vi "SVG Scale Example.vi"() -> ()   [LabVIEW 2020]
doc: "G-Image example demonstrating loading a vector image with adjustable scaling."
uses:
  <vilib>/picture/picture.llb/imagedata.ctl
  <vilib>/Utility/miscctls.llb/LVPointTypeDef.ctl
  Image IO/Polymorphic VIs/Load SVG Image (Path).vi
  <vilib>/Utility/cursorutil.llb/Set Cursor (Icon Pict).vi
  G-Image.lvlib
panel:
  in  "Reset View":bool
  in  "Image":u16(ring) items=["vector-gradient.svg", "vector.svg"]
  in  "Stop":bool
  out "2D Picture":picture
  in  "Scale":dbl(slide)=1.0 min=0.1 max=4.0 step=0.1 scale=0.1..4.0
  # "Instructions:\n1. Run the VI.\n2. Select a vector image to scale from the Image ring. \n3. Adjust the Scale slider to change the size of the vector image as it is loaded.\n4. Click and drag the image to pan the view. Reset the view by clicking Reset View."
  # "G"
  # "-Image"
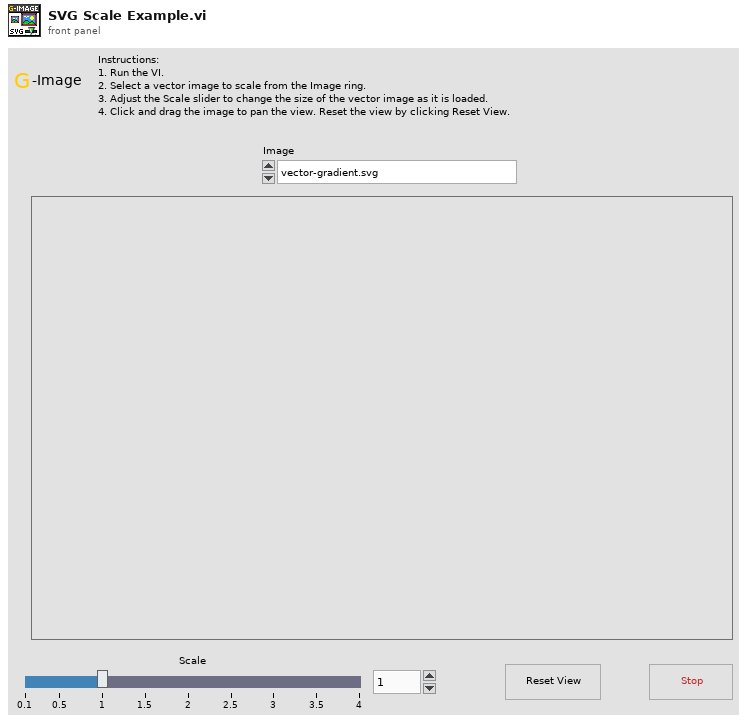
[diagram p1: front panel]
types:
  T1 = typedef "imagedata.ctl" = cluster{"image type":i32, "image depth":i32, "image":u8[], "mask":u8[], "colors":u32[], "Rectangle":cluster{"left":i16, "top":i16, "right":i16, "bottom":i16}}
  T2 = typedef "LVPoint32TypeDef.ctl" = cluster{"Horizontal":i32, "Vertical":i32}
  T3 = typedef "LVPointTypeDef.ctl" = cluster{"Horizontal":i16, "Vertical":i16}
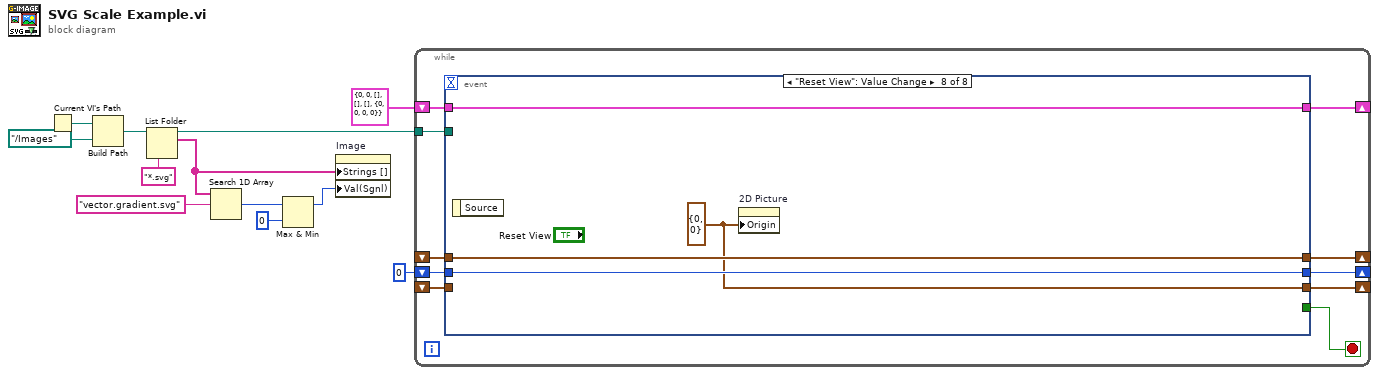
[diagram p0: block diagram]
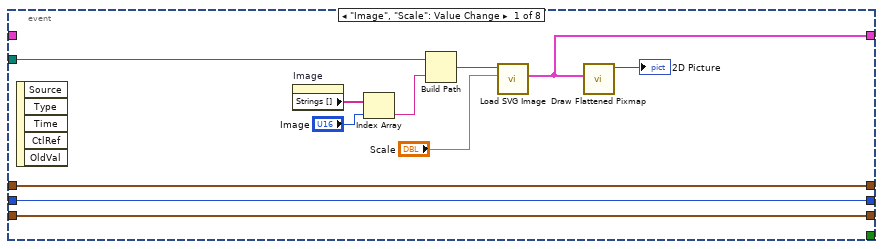
[diagram p2: hidden frame]
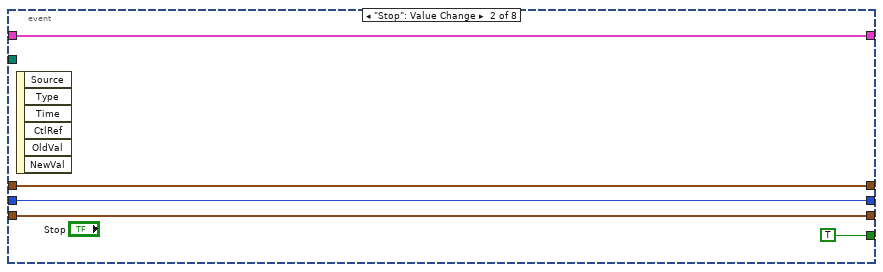
[diagram p3: hidden frame]
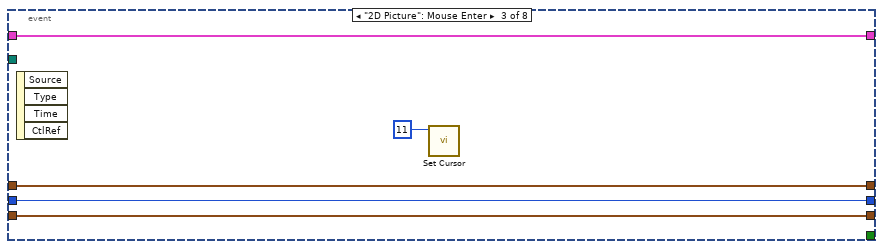
[diagram p4: hidden frame]
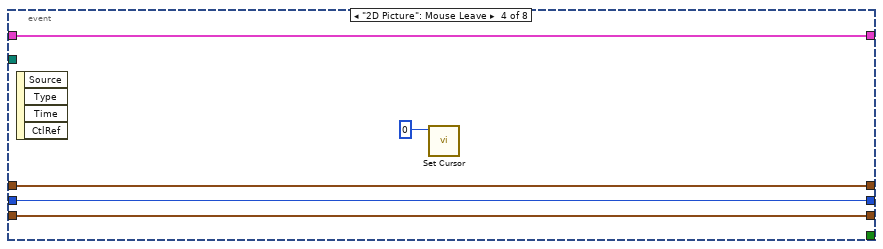
[diagram p5: hidden frame]
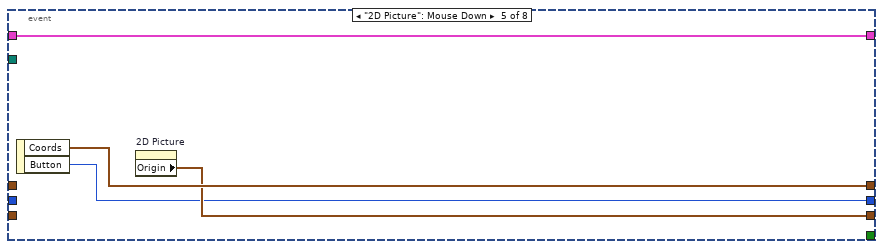
[diagram p6: hidden frame]
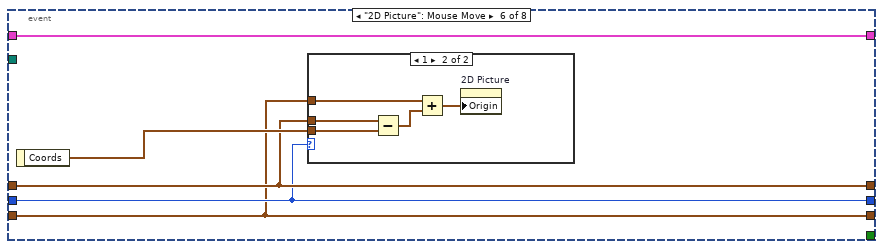
[diagram p7: hidden frame]
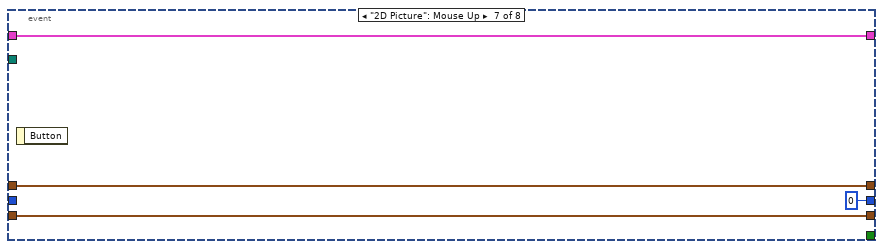
[diagram p9: hidden frame]
diagram:
  n1 = Current VI's Path() -> (path=w12:path)
  n2 = Build Path(base path=w12, name or relative path=path "../Images") -> (appended path=w10:path)
  n3 = List Folder(path=w10, pattern="*.svg") -> (path out=w9:path, filenames=w7:string[])  [unwired: 2 in, 2 out]
  n4 = Search 1D Array(1D array=w7, element="vector.gradient.svg") -> (index of element=w5:i32)  [unwired: 1 in]
  n5 = Max & Min(x=w5, y=0) -> (max(x,y)=w3:i32)  [unwired: 1 out]
  n6 = property on="Image" class="Ring (strict)"("Strings []"=w7, "Val(Sgnl)"=w3) -> ()  [unwired: 2 in, 2 out]
  n7 = while {
    tunnel: w9 -> [w20]
    shift-right: [w19] -> _
    shift-left: T1 {"image type"=0, "image depth"=0, "image"=[], "mask"=[], "colors"=[], "Rectangle"={"left"=0, "top"=0, "right"=0, "bottom"=0}} ("Image") -> [w22]
    shift-right: [w18] -> _
    shift-left: _ -> [w14]
    shift-right: [w17] -> _
    shift-left: _ -> [w16]
    shift-right: [w15] -> _
    shift-left: u16 0 ("Button") -> [w13]
    stop <- w21 stop-if-true
    n8 = event shown="[7] \"Reset View\": Value Change" {
      selector: _ -> [_ _ _ _ _ _ _ _]
      dyn-events: _ -> [_ _ _ _ _ _ _ _]
      timeout: _ -> [_ _ _ _ _ _ _ _]
      tunnel: w22 -> [_ w37 w42 w47 w49 w53 w66 w70]
      tunnel: [_ TRUE _ _ _ _ _ _] -> w21
      tunnel: w20 -> [w33 _ _ _ _ _ _ _]
      tunnel: [w27 w37 w42 w47 w49 w53 w66 w70] -> w19
      tunnel: [w25 w36 w41 w46 w52 w56 w65 w69] -> w18
      tunnel: [w23 w34 w39 w44 w51 w54 w64 w67] -> w17
      tunnel: w16 -> [w23 w34 w39 w44 _ w54 w64 _]
      tunnel: [w24 w35 w40 w45 w50 w55 u16 0 ("Button") w68] -> w15
      tunnel: w14 -> [w25 w36 w41 w46 _ w56 w65 w69]
      tunnel: w13 -> [w24 w35 w40 w45 _ w55 _ w68]
      event "Image", "Scale": Value Change {
        n9 = event-data() -> ()  [unwired: 1 in, 5 out]
        n10 = property on="Image" class="Ring (strict)"() -> ("Strings []"=w32:string[])  [unwired: 2 in, 2 out]
        n11 = Index Array(array=w32, index="Image") -> (element=w30:string)
        n12 = Build Path(base path=w33, name or relative path=w30) -> (appended path=w29:path)
        n13 = call-poly "Load SVG Image.vi"("Scale (1)"="Scale", "Path In"=w29) -> ("Image"=w27:T1)  [unwired: 7 in, 2 out]
        n14 = call <vilib>:"Draw Flattened Pixmap.vi"("image data"=w27) -> ("new picture"=→"2D Picture":picture)  [unwired: 8 in]
      }
      event "Stop": Value Change {
        n15 = event-data() -> ()  [unwired: 1 in, 6 out]
      }
      event "2D Picture": Mouse Enter {
        n16 = event-data() -> ()  [unwired: 1 in, 4 out]
        n17 = call-poly <vilib>:"Set Cursor.vi"("icon"=u16 11) -> ()  [unwired: 9 in, 2 out]
      }
      event "2D Picture": Mouse Leave {
        n18 = event-data() -> ()  [unwired: 1 in, 4 out]
        n19 = call-poly <vilib>:"Set Cursor.vi"("icon"=u16 0) -> ()  [unwired: 9 in, 2 out]
      }
      event "2D Picture": Mouse Down {
        n20 = event-data() -> ("Coords"=w52:T2, "Button"=w50:u16)  [unwired: 1 in]
        n21 = property on="2D Picture" class="Pict"() -> ("Origin"=w51:T3)  [unwired: 2 in, 2 out]
      }
      event "2D Picture": Mouse Move {
        n22 = event-data() -> ("Coords"=w57:T2)  [unwired: 1 in]
        n23 = case shown="1" w55 {
          tunnel: w57 -> [_ w62]
          tunnel: w56 -> [_ w61]
          tunnel: w54 -> [_ w59]
          frame 0, Default {
          }
          frame 1 {
            n24 = Subtract(x=w61, y=w62) -> (x-y=w60:T2)
            n25 = Add(x=w59, y=w60) -> (x+y=w58:T2)
            n26 = property on="2D Picture" class="Pict"("Origin"=w58) -> ()  [unwired: 2 in, 2 out]
          }
        }
      }
      event "2D Picture": Mouse Up {
        n27 = event-data() -> ()  [unwired: 1 in, 1 out]
      }
      event "Reset View": Value Change {
        w67 = T3 {"Horizontal"=0, "Vertical"=0} ("Origin")
        n28 = event-data() -> ()  [unwired: 1 in, 1 out]
        n29 = property on="2D Picture" class="Pict"("Origin"=w67) -> ()  [unwired: 2 in, 2 out]
      }
    }
  }
